vi "solar Msg UE Main Generate.vi"(4 "DATA Array":variant[](array[variant]), 6 "MSG Array":string[](array[string]), 7 "Priority? (F)":bool, 8 "error in (no error)":errorcluster, 9 "DATA (last)":variant, 10 "MSG (last)":string, 11 "solar in":refnum<class "solar.lvclass">) -> (0 "error out":errorcluster, 3 "solar out":refnum<class "solar.lvclass">)   [LabVIEW 2018]
doc: "This VI generates a User Event. If the message string is empty the a user event is not generated. The CMDs string array only writes to the CMD field. Set Priority to true to generate a priority user event."
uses:
  solar.lvclass
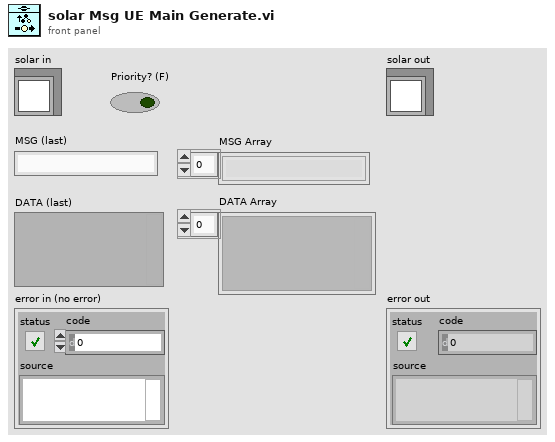
[diagram p1: front panel]
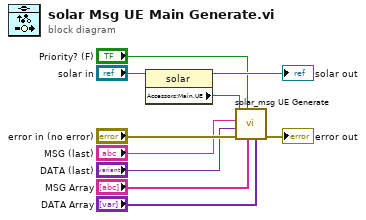
[diagram p0: block diagram]
diagram:
  n1 = property class="solar"(reference="solar in") -> (reference out=→"solar out":refnum<class "solar.lvclass">, "Accessors:Main.UE"=w6:refnum<user-event>)  [unwired: 1 in, 1 out]
  n2 = call "solar_msg UE Generate.vi"("CMD_DATA (Array)"="DATA Array", "CMD (Array)"="MSG Array", "Priority? (F)"="Priority? (F)", "error in (no error)"="error in (no error)", "CMD_DATA (Last)"="DATA (last)", "CMD (Last)"="MSG (last)", "UserEvent in"=w6) -> ("error out"=→"error out":errorcluster)  [unwired: 3 in, 1 out]
